vi "Calculate Playback Speed.vi"(9 "Pitch Bend Up (F)":bool, 10 "Pitch Bend Down (F)":bool, 11 "Pitch":dbl) -> (3 "Speed Multiplier":dbl)   [LabVIEW 2018, in "Audio Processing.lvlib"]
doc: "Convert pitch (-30 to 30) into speed multiplier (0.7 to 1.3), with adjustments made for pitch bending."
uses:
  Audio Processing.lvlib
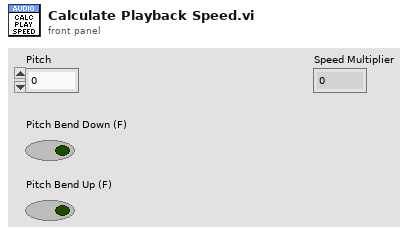
[diagram p1: front panel]
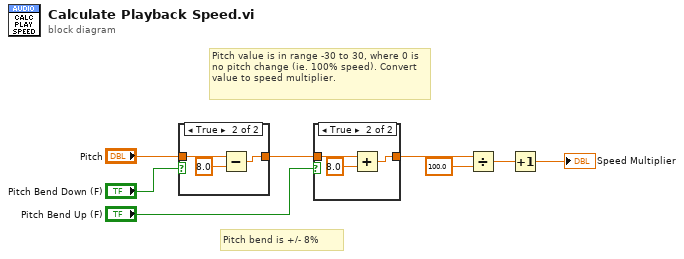
[diagram p0: block diagram]
diagram:
  # "Pitch bend is +/- 8%"
  # "Pitch value is in range -30 to 30, where 0 is no pitch change (ie. 100% speed). Convert value to speed multiplier."
  n1 = case shown="True" "Pitch Bend Down (F)" {
    tunnel: "Pitch" -> [w9 w12]
    tunnel: [w9 w10] -> w6
    frame False {
    }
    frame True {
      n2 = Subtract(x=w12, y=8.0) -> (x-y=w10:dbl)
    }
  }
  n3 = case shown="True" "Pitch Bend Up (F)" {
    tunnel: w6 -> [w13 w16]
    tunnel: [w13 w14] -> w5
    frame False {
    }
    frame True {
      n4 = Add(x=w16, y=8.0) -> (x+y=w14:dbl)
    }
  }
  n5 = Divide(x=w5, y=100.0) -> (x/y=w7:dbl)
  n6 = Increment(x=w7) -> (x+1=→"Speed Multiplier":dbl)
